vi "Read Server Configuration.vi"(8 "error in (no error)":errorcluster) -> (0 "error out":errorcluster)   [LabVIEW 2024]
doc: "Reads the server configuration from configuration files. The server configuration includes system configuration and subsystem I/O attributes configuration."
uses:
  Controls/Server/System Configuration.ctl
  Controls/Server/Subsystem Configuration.ctl
  Controls/Server/Subsystem IO Attributes.ctl
  Controls/Server/Subsystem IO Logging Attributes.ctl
  Controls/Server/Subsystem IO Alarm Attributes.ctl
  Globals/Global - Server.vi
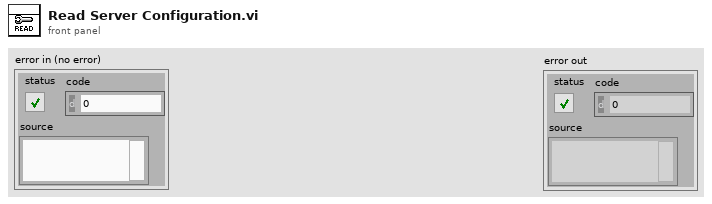
[diagram p1: front panel]
types:
  T1 = typedef "Subsystem IO Attributes.ctl" = cluster{"Name":string, "Data Type":enum32{"u32BitField", "bool", "double", "string", "int8", "uint8", "int16", "uint16", "int32", "uint32", "int64", "uint64", "single", "double waveform", "int16 waveform", "array of boolean", "array of int8", "array of uint8", "array of int16", "array of uint16", "array of int32", "array of uint32", "array of int64", "array of uint64", "array of single", "array of double", "array of double waveform", "array of int16 waveform", "array of string", "variant", "timestamp", "fixed point", "custom"}, "Access Type":enum32{"Read only", "Write only", "Read/write"}, "Alarm Enabled?":bool, "Logging Enabled?":bool, "Logging Attributes":T2, "Alarm Attributes":T3}
  T2 = typedef "Subsystem IO Logging Attributes.ctl" = cluster{"log data? (F)":bool, "log alarms & events? (F)":bool}
  T3 = typedef "Subsystem IO Alarm Attributes.ctl" = cluster{"Hi:enable? (F)":bool, "Hi:name":string, "Hi:level/change":dbl, "Lo:enable? (F)":bool, "Lo:name":string, "Lo:level/change":dbl, "Boolean:enable? (F)":bool, "Boolean:name":string, "Boolean:value":bool, "BadStatus:enable? (F)":bool, "BadStatus:name":string}
  T4 = typedef "System Configuration.ctl" = cluster{"Name":string, "Description":string, "Logging Computer Name":string, "Logging Database Name":string, "Logging Database Path":path, "Archive Computer Name":string, "Archive Database Name":string, "Archive Database Path":path, "Lifespan (days)":u32, "Archive Enabled":bool, "Archive Interval (hours)":u32, "Subsystems":T5[]}
  T5 = typedef "Subsystem Configuration.ctl" = cluster{"Name":string, "Root URL":refnum<k21>}
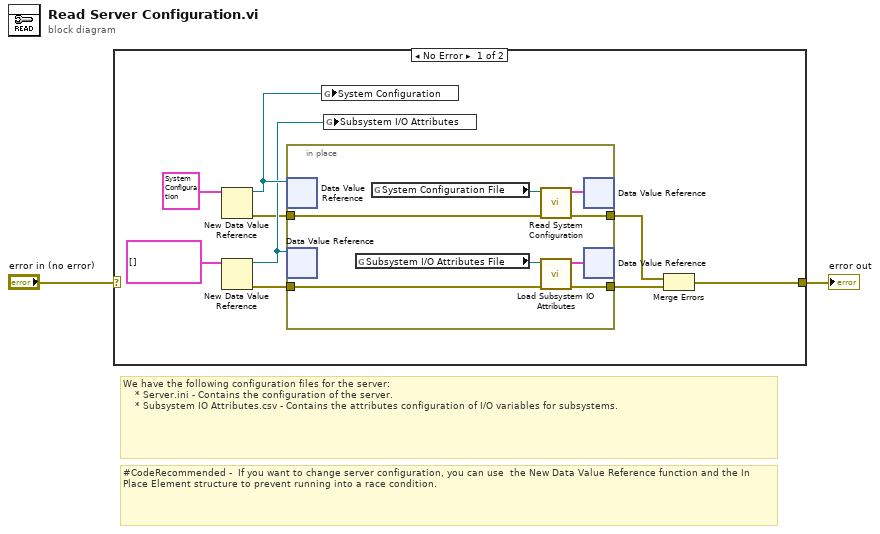
[diagram p0: block diagram]
diagram:
  # "#CodeRecommended -  If you want to change server configuration, you can use  the New Data Value Reference function and the In Place Element structure to prevent running into a race condition."
  # "We have the following configuration files for the server:\n    * Server.ini - Contains the configuration of the server.\n    * Subsystem IO Attributes.csv - Contains the attributes configuration of I/O variables for subsystems."
  n1 = case shown="No Error" "error in (no error)" {
    selector: "error in (no error)" -> [_ w20]
    tunnel: [w9 w20] -> w1
    frame No Error {
      n2 = New Data Value Reference(data value=T4 {"Name"="", "Description"="", "Logging Computer Name"="", "Logging Database Name"="", "Logging Database Path"=path "", "Archive Computer Name"="", "Archive Database Name"="", "Archive Database Path"=path "", "Lifespan (days)"=0, "Archive Enabled"=FALSE, "Archive Interval (hours)"=0, "Subsystems"=[]} ("System Configuration")) -> (data value reference=w6:refnum<data-value>, error out=w3:errorcluster)  [unwired: 1 in]
      n3 = New Data Value Reference(data value=T1[] []) -> (data value reference=w5:refnum<data-value>, error out=w4:errorcluster)  [unwired: 1 in]
      n4 = in-place {
        in-place-border: [w16] -> w8
        in-place-border: [w14] -> w7
        in-place-border: w4 -> [w13]
        in-place-border: w3 -> [w12]
        n5 = in-place-dvr #1(w6) -> ()  [unwired: 2 out]
        n6 = in-place-dvr #2(w5) -> ()  [unwired: 2 out]
        n7 = global read "Global - Server.vi" "Subsystem I/O Attributes File"() -> (w18:path)
        n8 = global read "Global - Server.vi" "System Configuration File"() -> (w19:path)
        n9 = call "Read System Configuration.vi"("error in (no error)"=w12, "System Configuration File Path"=w19) -> ("error out"=w16:errorcluster, "System Configuration"=w17:T4)  [unwired: 8 in]
        n10 = call "Load Subsystem IO Attributes.vi"("error in (no error)"=w13, "Subsystem I/O Attributes File Path"=w18) -> ("error out"=w14:errorcluster, "Subsystem I/O Attributes"=w15:T1[])  [unwired: 8 in]
        n11 = in-place-dvr #1(w17) -> ()  [unwired: 2 out]
        n12 = in-place-dvr #2(w15) -> ()  [unwired: 2 out]
      }
      n13 = global write "Global - Server.vi" "System Configuration"(w6) -> ()
      n14 = global write "Global - Server.vi" "Subsystem I/O Attributes"(w5) -> ()
      n15 = Merge Errors(w8, w7) -> (w9:errorcluster)
    }
    frame Error {
    }
  }
  "error out" <- w1
